vi "Register.vi"(8 "error in":errorcluster, 10 "TPCANHandle":T1 items=["PCAN_NONEBUS"=0, "PCAN_USBBUS1"=81, "PCAN_USBBUS2"=82, "PCAN_USBBUS3"=83, "PCAN_USBBUS4"=84, "PCAN_USBBUS5"=85, "PCAN_USBBUS6"=86, "PCAN_USBBUS7"=87, "PCAN_USBBUS8"=88, "PCAN_USBBUS9"=1289, "PCAN_USBBUS10"=1290, "PCAN_USBBUS11"=1291, "PCAN_USBBUS12"=1292, "PCAN_USBBUS13"=1293, "PCAN_USBBUS14"=1294, "PCAN_USBBUS15"=1295, "PCAN_USBBUS16"=1296], 11 "epoll in":refnum<class "epoll.lvclass">) -> (0 "error out":errorcluster, 3 "epoll out":refnum<class "epoll.lvclass">)   [LabVIEW 2020, in "PCANBasic.lvlib" / "epoll.lvclass"]
uses:
  epoll.lvclass
  epoll.lvclass/epoll.ctl
  PCANBasic.lvlib
  Get Receive Event.vi
  TPCANHandle.ctl
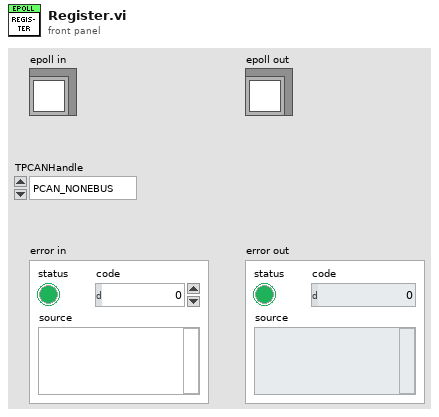
[diagram p1: front panel]
types:
  T1 = typedef "PCANBasic.lvlib/TPCANHandle.ctl" = u16
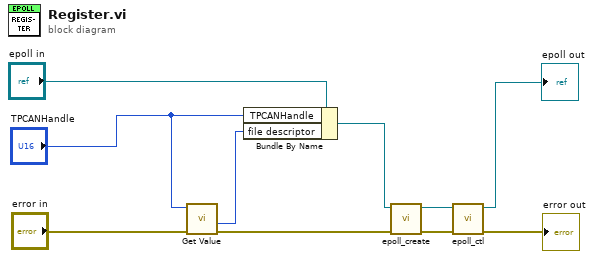
[diagram p0: block diagram]
diagram:
  n1 = call-poly "Get Value.vi"("error in"="error in", "TPCANHandle in"="TPCANHandle") -> ("error out"=w9:errorcluster, "Filedescriptor fd (Linux)"=w7:i32)  [unwired: 5 in, 3 out]
  n2 = Bundle By Name(cluster="epoll in", "TPCANHandle"="TPCANHandle", "file descriptor"=w7) -> (w4:refnum<class "epoll.lvclass">)
  n3 = call "epoll_create.vi"("error in"=w9, "epoll in"=w4) -> ("error out"=w5:errorcluster, "epoll out"=w2:refnum<class "epoll.lvclass">)  [unwired: 8 in]
  n4 = call "epoll_ctl.vi"("error in"=w5, "epoll in"=w2) -> ("error out"=→"error out":errorcluster, "epoll out"=→"epoll out":refnum<class "epoll.lvclass">)  [unwired: 8 in]
